vi "Set Queue ACL.vi"(8 "error in (no error)":errorcluster, 9 "ACL":T1[](array[typedef]), 10 "Queue":string, 11 "Azure Session in":refnum<class "Session.lvclass">) -> (0 "error out":errorcluster, 3 "Azure Session out":refnum<class "Session.lvclass">)   [LabVIEW 2015, in "NI_Azure_Queue.lvlib"]
doc: "Sets stored access policies for the queue that may be used with Shared Access Signatures."
uses:
  NI_Azure_Queue.lvlib
  Core/Session/Session.lvclass
  Signed Identifier.ctl
  Access Policy.ctl
  Core/Name Value Pair.ctl
  Core/Session/Session.lvclass/Session.ctl
  Core/Session/Write Request Parameters.vi
  Core/Session/Write Request body.vi
  Core/Session/Write HTTP Verb.vi
  Core/Session/Write URL Suffix.vi
  Core/NI_Azure_Core.lvlib
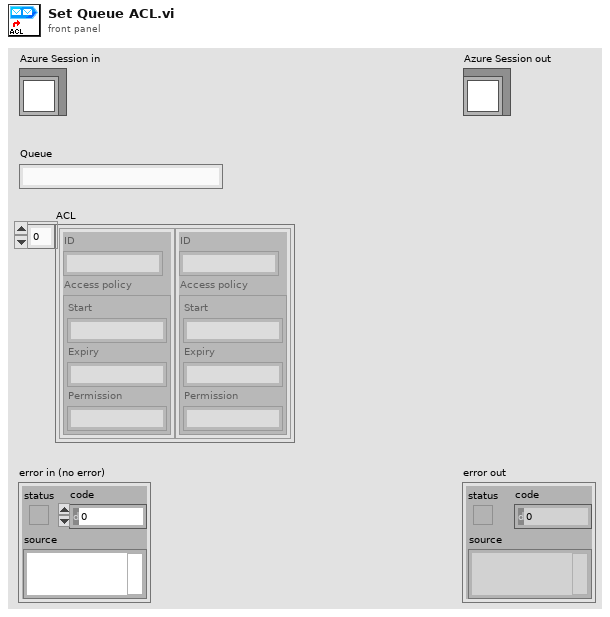
[diagram p1: front panel]
types:
  T1 = typedef "NI_Azure_Queue.lvlib/Signed Identifier.ctl" = cluster{"ID":string, "Access policy":T2}
  T2 = typedef "NI_Azure_Queue.lvlib/Access Policy.ctl" = cluster{"Start":string, "Expiry":string, "Permission":string}
  T3 = typedef "NI_Azure_Core.lvlib/Name Value Pair.ctl" = cluster{"name":string, "value":string}
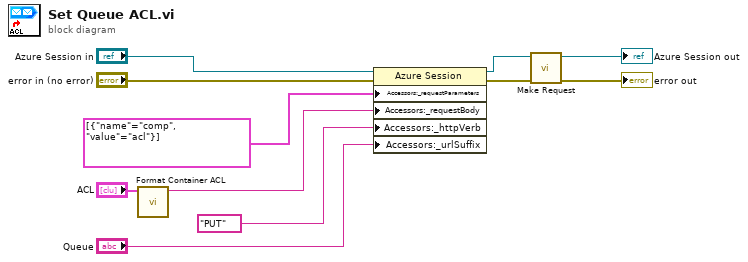
[diagram p0: block diagram]
diagram:
  n1 = call "Format Container ACL.vi"("ACL"="ACL") -> ("ACL string"=w4:string)  [unwired: 10 in]
  n2 = property class="Azure Session"(reference="Azure Session in", error in="error in (no error)", "Accessors:_requestParameters"=T3[] [{"name"="comp", "value"="acl"}] ("request parameters"), "Accessors:_requestBody"=w4, "Accessors:_httpVerb"="PUT" ("HTTP-Verb"), "Accessors:_urlSuffix"="Queue") -> (reference out=w7:refnum<class "Session.lvclass">, error out=w5:errorcluster)
  n3 = call "Make Request.vi"("error in (no error)"=w5, "Session in"=w7) -> ("error out"=→"error out":errorcluster, "Session out"=→"Azure Session out":refnum<class "Session.lvclass">)  [unwired: 7 in, 1 out]
